vi "CANOpen_SDO Report Error to Console.vi"(6 "Caller":string, 7 "Node ID":u8, 8 "error in (no error)":errorcluster, 9 "Object Sub-Index":u8, 10 "Object Index":u16, 11 "completion code":u32) -> ()   [LabVIEW 2021, in "CANOpen Addon Engine.lvlib"]
uses:
  CANOpen Addon Engine.lvlib
  <vilib>/NI VeriStand/Custom Device Tools/Custom Device Utility Library/RT Debug String Color Spec.ctl
  <vilib>/NI VeriStand/Custom Device Tools/Custom Device Utility Library/Custom Device Utility Library.lvlib
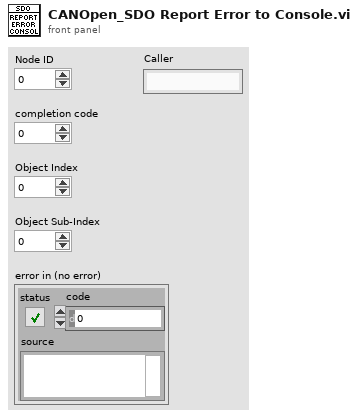
[diagram p1: front panel]
types:
  T1 = typedef "Custom Device Utility Library.lvlib/RT Debug String Color Spec.ctl" = u16
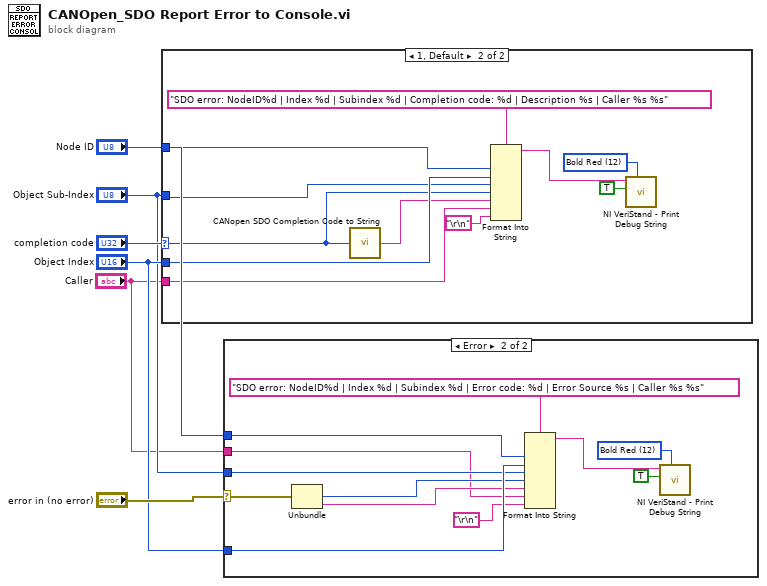
[diagram p0: block diagram]
diagram:
  n1 = case shown="1, Default" "completion code" {
    selector: "completion code" -> [_ w10]
    tunnel: "Node ID" -> [_ w14]
    tunnel: "Object Sub-Index" -> [_ w11]
    tunnel: "Object Index" -> [_ w12]
    tunnel: "Caller" -> [_ w8]
    frame 0 {
    }
    frame 1, Default {
      w17 = T1 12 items=["Plain White"=7, "Bold White"=15, "Bold Blue"=9, "Bold Green"=10, "Bold Red"=12] ("Attribute")
      n2 = call <vilib>:"CANopen SDO Completion Code to String.vi"("SDO completion code"=w10) -> ("description"=w9:string)
      n3 = Format Into String(format string="SDO error: NodeID%d | Index %d | Subindex %d | Completion code: %d | Description %s | Caller %s %s", w14, w12, w11, w10, w9, w8, "\r\n") -> (resulting string=w13:string)  [unwired: 2 in, 1 out]
      n4 = call <vilib>:"NI VeriStand - Print Debug String.vi"("Attribute"=w17, "Add to log file? (F)"=TRUE ("Add to log file? (T)"), "Message"=w13) -> ()  [unwired: 8 in, 1 out]
    }
  }
  n5 = case shown="Error" "error in (no error)" {
    selector: "error in (no error)" -> [_ w29]
    tunnel: "Node ID" -> [_ w24]
    tunnel: "Object Index" -> [_ w23]
    tunnel: "Object Sub-Index" -> [_ w22]
    tunnel: "Caller" -> [_ w19]
    frame No Error {
    }
    frame Error {
      w25 = T1 12 items=["Plain White"=7, "Bold White"=15, "Bold Blue"=9, "Bold Green"=10, "Bold Red"=12] ("Attribute")
      n6 = Unbundle(w29) -> ("code"=w21:i32, "source"=w20:string)  [unwired: 1 out]
      n7 = Format Into String(format string="SDO error: NodeID%d | Index %d | Subindex %d | Error code: %d | Error Source %s | Caller %s %s", w24, w23, w22, w21, w20, w19, "\r\n") -> (resulting string=w28:string)  [unwired: 2 in, 1 out]
      n8 = call <vilib>:"NI VeriStand - Print Debug String.vi"("Attribute"=w25, "Add to log file? (F)"=TRUE ("Add to log file? (T)"), "Message"=w28) -> ()  [unwired: 8 in, 1 out]
    }
  }
